vi "ExpectationFailedError.vi"(7 "Source (caller)":string, 8 "error in (no error)":errorcluster, 10 "Message":string) -> (0 "error out":errorcluster)   [LabVIEW 2017, in "Error.lvlib"]
doc: "Creates an error with error code <B>-8000</B>. Optionally accepts an error <B>source</B> to replace the caller's VI name in the error message. Use for constraints that failed their expectation.\n\nIf an error is detected at the <B>error in</B> terminal, the error is passed to the <B>error out</B> terminal."
uses:
  Error.lvlib
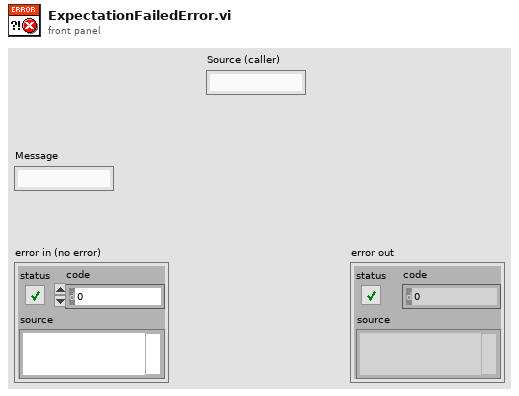
[diagram p1: front panel]
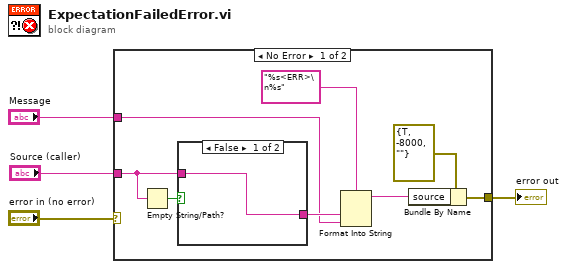
[diagram p0: block diagram]
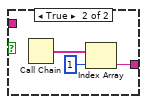
[diagram p2: hidden frame]
diagram:
  n1 = case shown="No Error" "error in (no error)" {
    selector: "error in (no error)" -> [_ w17]
    tunnel: [w11 w17] -> w4
    tunnel: "Message" -> [w7 _]
    tunnel: "Source (caller)" -> [w5 _]
    frame No Error {
      n2 = Empty String/Path?(string/path=w5) -> (empty?=w6:bool)
      n3 = case shown="False" w6 {
        tunnel: [w13 w15] -> w8
        tunnel: w5 -> [w13 _]
        frame False {
        }
        frame True {
          n4 = Call Chain() -> (call chain=w16:string[])
          n5 = Index Array(array=w16, index=1) -> (element=w15:string)
        }
      }
      n6 = Format Into String(format string="%s<ERR>\n%s", w8, w7) -> (resulting string=w9:string)  [unwired: 2 in, 1 out]
      n7 = Bundle By Name(cluster=errorcluster {"status"=TRUE, "code"=-8000, "source"=""} ("error constant"), "source"=w9) -> (w11:errorcluster)
    }
    frame Error {
    }
  }
  "error out" <- w4
